vi "Remove Item.vi"(8 "error in (no error)":errorcluster, 11 "SE UI cluster in":T1={"Node Ptr"=18446744073709551615, "Add"=refnum, "Remove"=refnum, "Registers ListBox"=refnum} {"Node Ptr" format="%.0x"}) -> (0 "error out":errorcluster, 2 "Deleted?":bool, 3 "SE UI cluster out":T1={"Node Ptr"=18446744073709551615, "Add"=refnum, "Remove"=refnum, "Registers ListBox"=refnum} {"Node Ptr" format="%.0x"})   [LabVIEW 2020, in "FPGA Addon System Explorer.lvlib"]
uses:
  FPGA Addon System Explorer.lvlib
  Types/SE UI Cluster.ctl
  <vilib>/NI VeriStand/Custom Device API/Custom Device Item Ref.ctl
  <vilib>/NI VeriStand/Custom Device API/Custom Device API.lvlib
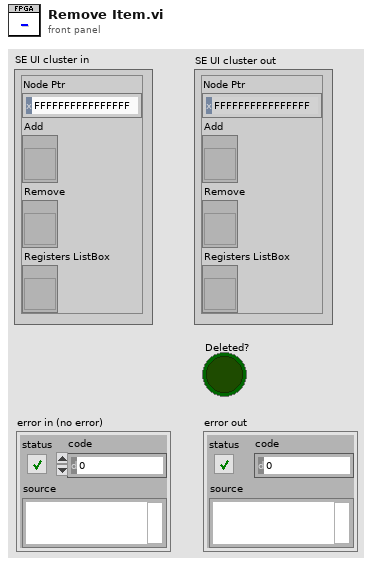
[diagram p1: front panel]
types:
  T1 = typedef "FPGA Addon System Explorer.lvlib/SE UI Cluster.ctl" = cluster{"Node Ptr":T2, "Add":refnum<vi>, "Remove":refnum<vi>, "Registers ListBox":refnum<vi>}
  T2 = typedef "Custom Device API.lvlib/Custom Device Item Ref.ctl" = u64
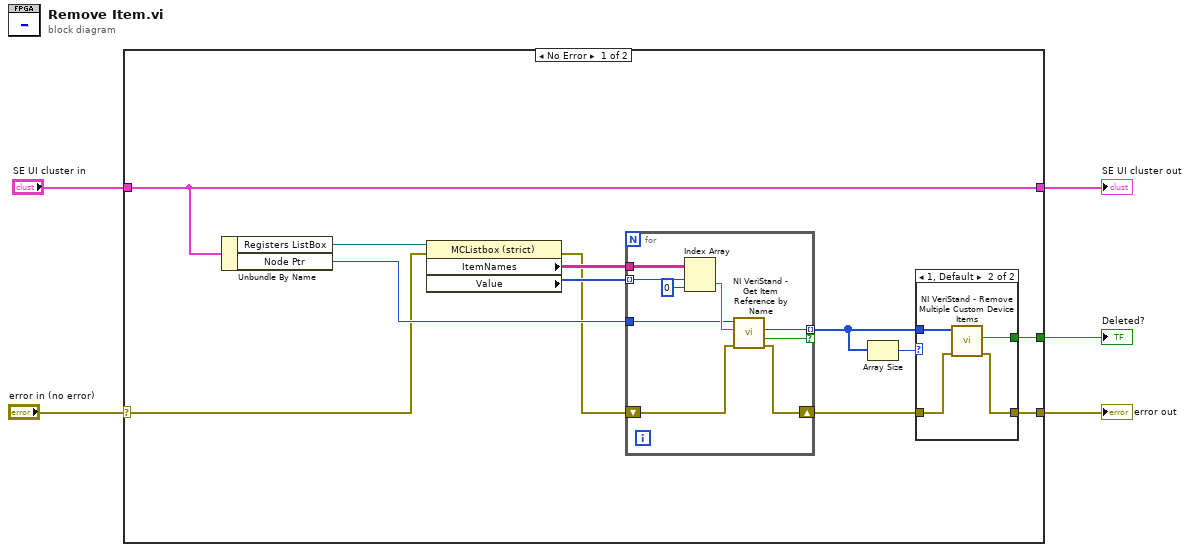
[diagram p0: block diagram]
diagram:
  n1 = case shown="No Error" "error in (no error)" {
    selector: "error in (no error)" -> [w13 w33]
    tunnel: "SE UI cluster in" -> [w9 w32]
    tunnel: [w10 w33] -> w3
    tunnel: [w9 w32] -> w2
    tunnel: [w8 _] -> w1
    frame No Error {
      n2 = Unbundle By Name(w9) -> ("Registers ListBox"=w17:refnum<vi>, "Node Ptr"=w14:T2)
      n3 = property class="MCListbox (strict)"(reference=w17, error in=w13) -> (error out=w12:errorcluster, "ItemNames"=w16:string[][], "Value"=w15:i32[])  [unwired: 1 out]
      n4 = for {
        tunnel: w16 -> [w31]
        tunnel: w15 -> [w30] mode=indexing
        tunnel: w14 -> [w27]
        tunnel: [w26] -> w7 mode=indexing if=w25
        shift-right: [w23] -> w11
        shift-left: w12 -> [w24]
        n5 = Index Array(array=w31, index (row)=w30, index (col)=0 ("disabled index (col)")) -> (element=w29:string)
        n6 = call <vilib>:"NI VeriStand - Get Item Reference by Name.vi"("error in (no error)"=w24, "Item Name"=w29, "Parent Ref in"=w27) -> ("error out"=w23:errorcluster, "Item Ref"=w26:T2, "Found"=w25:bool)  [unwired: 5 in, 1 out]
      }
      n7 = Array Size(array=w7) -> (size(s)=w6:i32)
      n8 = case shown="1, Default" w6 {
        tunnel: w11 -> [w18 w22]
        tunnel: [w18 w21] -> w10
        tunnel: [_ w20] -> w8
        tunnel: w7 -> [_ w19]
        frame 0 {
        }
        frame 1, Default {
          n9 = call <vilib>:"NI VeriStand - Remove Multiple Custom Device Items.vi"("error in (no error)"=w22, "Item Refs in"=w19) -> ("error out"=w21:errorcluster, "Deleted?"=w20:bool)  [unwired: 8 in]
        }
      }
    }
    frame Error {
    }
  }
  "error out" <- w3
  "SE UI cluster out" <- w2
  "Deleted?" <- w1
